vi "midi_UniqueChannels.vi"(10 "channels":u8[](array[numeric])) -> (2 "channel list":string)   [LabVIEW 2013]
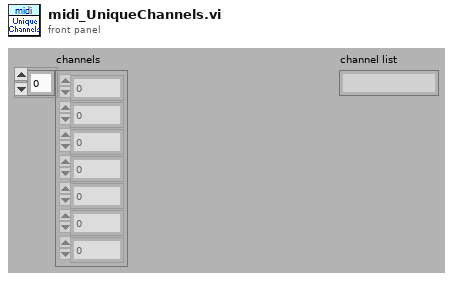
[diagram p1: front panel]
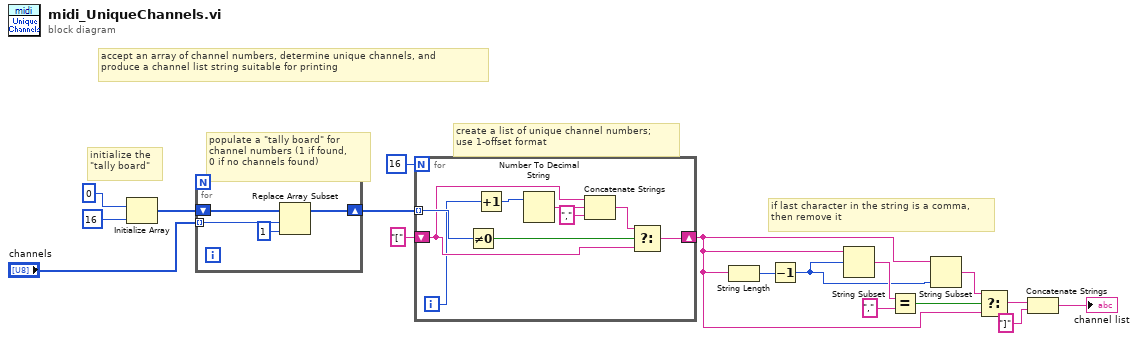
[diagram p0: block diagram]
diagram:
  # "if last character in the string is a comma,\nthen remove it"
  # "create a list of unique channel numbers;\nuse 1-offset format"
  # "populate a \"tally board\" for\nchannel numbers (1 if found,\n0 if no channels found)"
  # "initialize the\n\"tally board\""
  # "accept an array of channel numbers, determine unique channels, and\nproduce a channel list string suitable for printing"
  n1 = Initialize Array(u8 0 ("element"), 16 ("dimension size")) -> (w15:u8[])
  n2 = for {
    shift-right: [w20] -> w12
    shift-left: w15 -> [w21]
    tunnel: "channels" -> [w19] mode=indexing
    n3 = Replace Array Subset(array=w21, new element=u8 1 ("new element/subarray"), index=w19) -> (w20:u8[])
  }
  n4 = for {
    N: 16 -> [_]
    tunnel: w12 -> [w30] mode=indexing
    shift-right: [w28] -> w4
    shift-left: "[" ("f") -> [w24]
    i -> [w23]
    n5 = Not Equal To 0?(x=w30) -> (x != 0?=w29:bool)
    n6 = Increment(x=w23) -> (x+1=w22:i32)
    n7 = Number To Decimal String(number=w22) -> (decimal integer string=w27:string)  [unwired: 1 in]
    n8 = Concatenate Strings(w24, w27, "," ("string")) -> (w25:string)
    n9 = Select(t=w25, s=w29, f=w24) -> (s? t:f=w28:string)
  }
  n10 = String Length(string=w4) -> (length=w10:i32)
  n11 = Decrement(x=w10) -> (x-1=w6:i32)
  n12 = String Subset(string=w4, offset (0)=w6) -> (substring=w9:string)  [unwired: 1 in]
  n13 = Equal?(x=w9, y=",") -> (x = y?=w7:bool)
  n14 = String Subset(string=w4, length (rest)=w6) -> (substring=w5:string)  [unwired: 1 in]
  n15 = Select(t=w5, s=w7, f=w4) -> (s? t:f=w3:string)
  n16 = Concatenate Strings(w3, "]" ("string")) -> (→"channel list":string)
